vi "Waveform_Creator.vi"() -> ()   [LabVIEW 2012]
uses:
  Waveform.ctl
  Terminal_Control.vi
  <vilib>/Instr/_visa.llb/VISA Configure Serial Port (Instr).vi
panel:
  in  "COM Port":refnum<visa-resource-name>="COM3"
  in  "Terminal":i32(listbox)
  out "Active Port":refnum<visa-resource-name>
  in  "OPEN PORT":bool
  out "Waveform Library":T1[](array[typedef]) {"Envelope Shape" items=["SQUARE", "TRIANGLE", "SINE"]; "Envelope Duty Cycle" min=0.0 max=100.0 step=1.0; "Cos 1 Amplitude" min=0.0 max=100.0 step=1.0; "Cos 1 Frequency" min=0.0 max=100.0 step=0.1; "Cos 2 Amplitude" min=0.0 max=100.0 step=1.0; "Cos 2 Frequency" min=0.0 max=100.0 step=0.1}
  in  "Tab Control":enum32{"Waveform Design", "Motor Control"}(tab)
  in  "SAVE_LIBARY":bool
  in  "LOAD_LIBARY":bool
  in  "Waveform Object":T1={"Cos 2 Frequency"=2.0, "Cos 2 Amplitude"=50.0, "Cos 1 Frequency"=2.0, "Cos 1 Amplitude"=100.0, "Envelope Duty Cycle"=100.0, "Envelope Shape"=1} {"Envelope Shape" items=["SQUARE", "TRIANGLE", "SINE"]; "Envelope Duty Cycle" min=0.0 max=100.0 step=1.0; "Cos 1 Amplitude" min=0.0 max=100.0 step=1.0; "Cos 1 Frequency" min=0.0 max=100.0 step=0.1; "Cos 2 Amplitude" min=0.0 max=100.0 step=1.0; "Cos 2 Frequency" min=0.0 max=100.0 step=0.1}
  out "Waveform Graph":dbl[][](graph)
  out "Command":string="W(6,2,100,20,100,20,50)"
  in  "Program":bool
  in  "Waveform Slot":dbl=6.0 min=0.0 max=50.0 step=1.0
  in  "Run":bool[](array[boolean])=[FALSE, FALSE, FALSE, FALSE, FALSE, FALSE, TRUE, FALSE, FALSE, TRUE, FALSE, FALSE, FALSE, FALSE, FALSE, TRUE, FALSE]
  in  "Frequency_Array":dbl[](array[numeric])=[10.0, 10.0, 10.0, 10.0, 10.0, 10.0, 10.0, 10.0, 10.0, 10.0, 10.0, 10.0, 10.0, 10.0, 10.0, 10.0] caption="Frequency"
  in  "Amplitude_Array":dbl[](array[numeric])=[4095.0, 4095.0, 4095.0, 4095.0, 4095.0, 4095.0, 4095.0, 4095.0, 4095.0, 4095.0, 4095.0, 4095.0, 4095.0, 4095.0, 4095.0, 4095.0] caption="Amplitude"
  in  "Waveform Array":dbl[](array[numeric])=[0.0, 0.0, 0.0, 0.0, 0.0, 0.0, 3.0, 0.0, 0.0, 0.0, 0.0, 0.0, 0.0, 0.0, 0.0, 0.0] caption="Waveform"
  # "Amplitude"
  # "Frequency"
  # "COSINE 1"
  # "COSINE 2"
  # "Waveform Library"
  # "Amplitude"
  # "Frequency"
  # "COSINE 1"
  # "COSINE 2"
  # "Motor"
  # "1\n2\n3\n4\n5\n6\n7\n8\n9\n10\n11\n12\n13\n14\n15\n16"
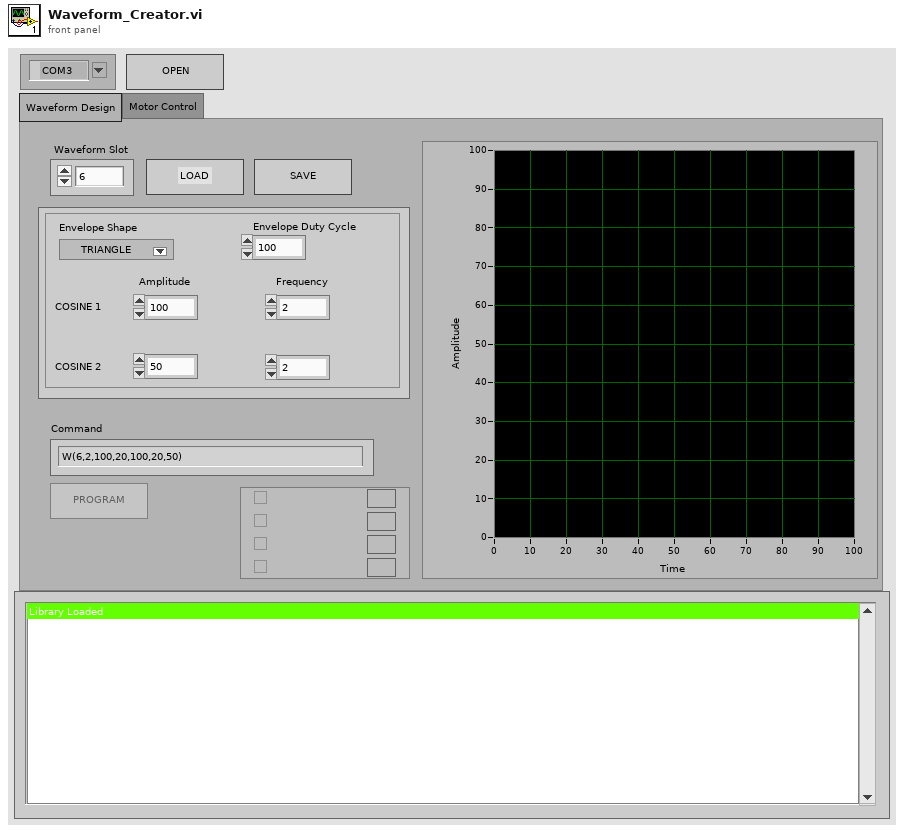
[diagram p1: front panel]
types:
  T1 = typedef "Waveform.ctl" = cluster{"Cos 2 Frequency":dbl, "Cos 2 Amplitude":dbl, "Cos 1 Frequency":dbl, "Cos 1 Amplitude":dbl, "Envelope Duty Cycle":dbl, "Envelope Shape":u16}
  T2 = enum8{"Enabled", "Disabled", "Disabled and Grayed Out"}
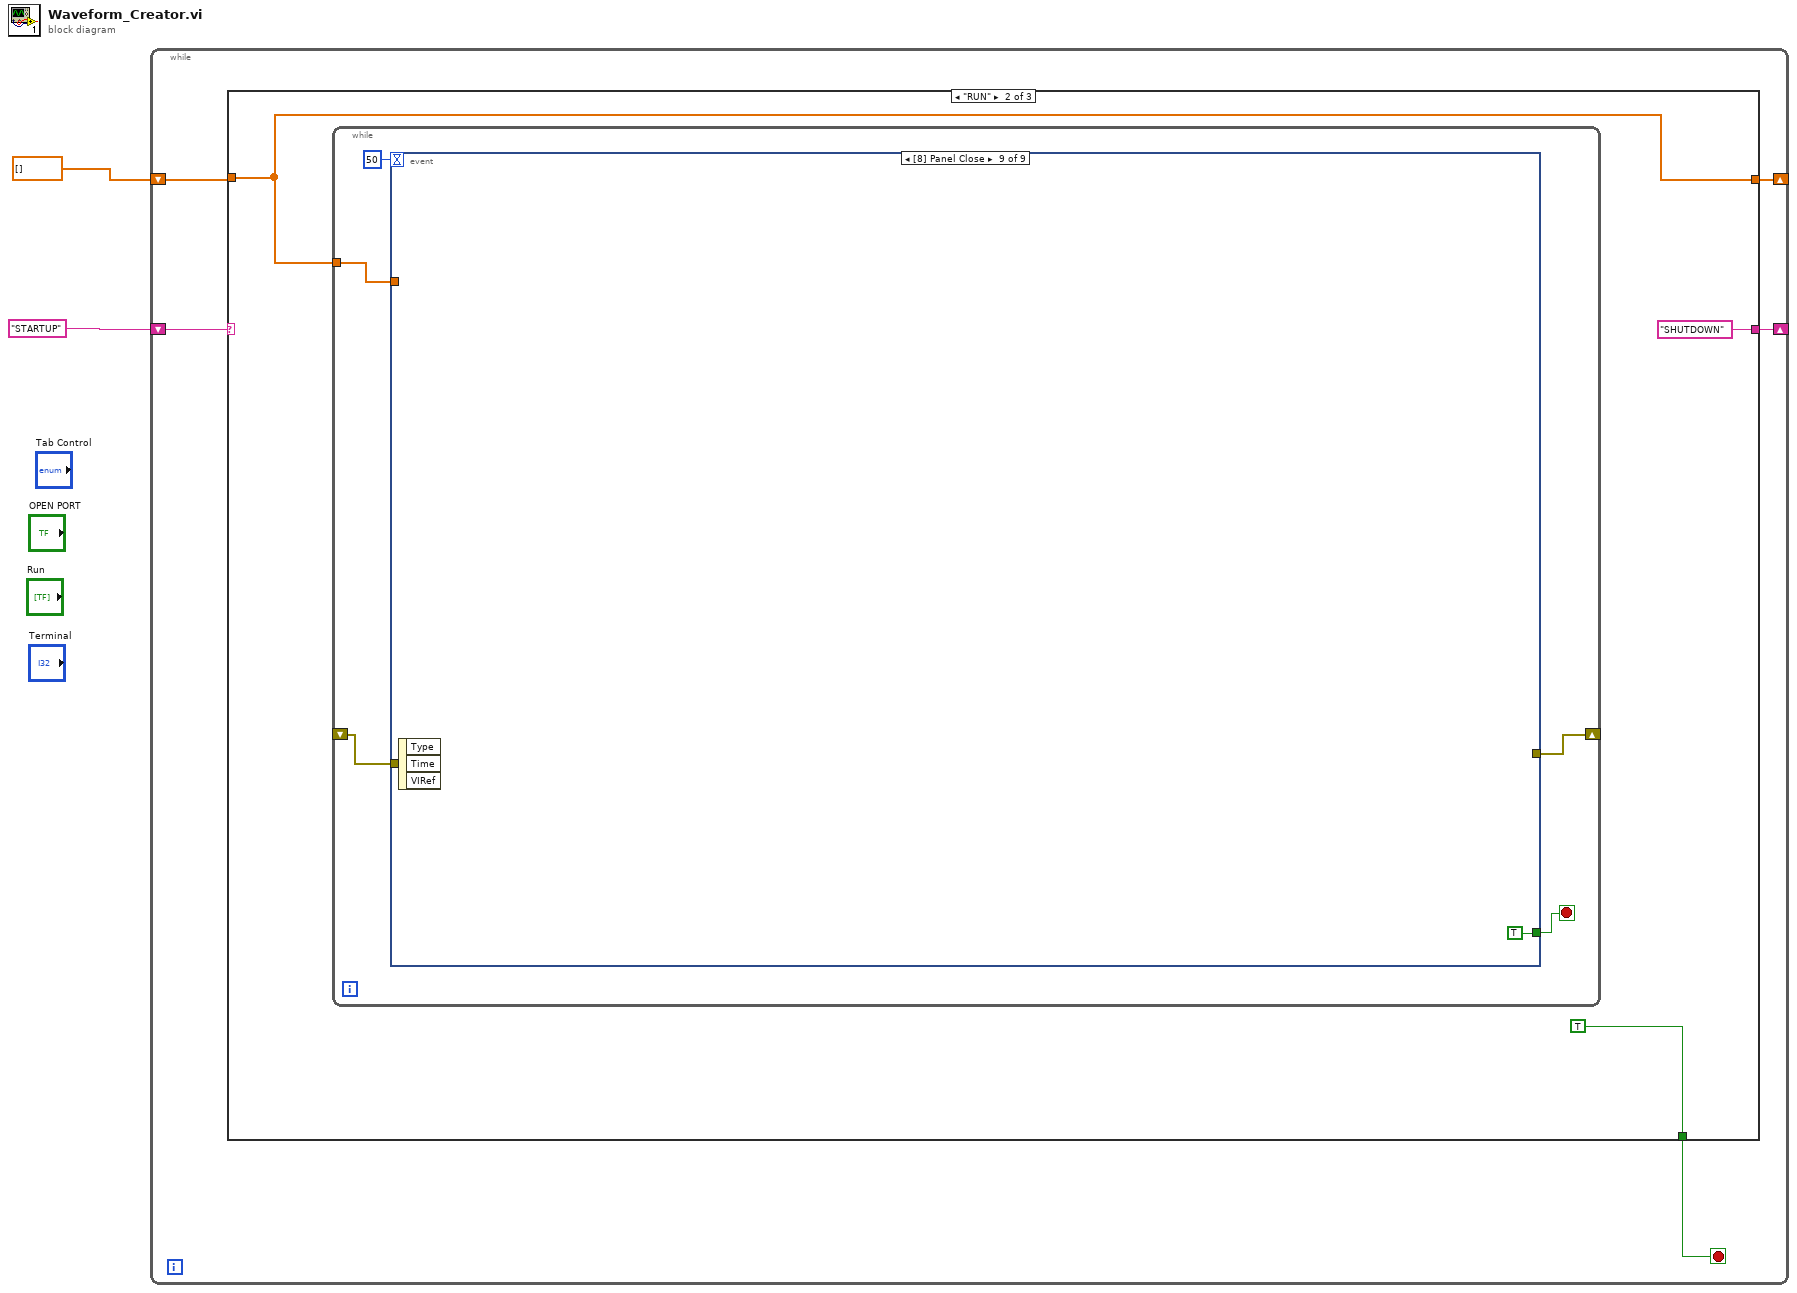
[diagram p0: block diagram]
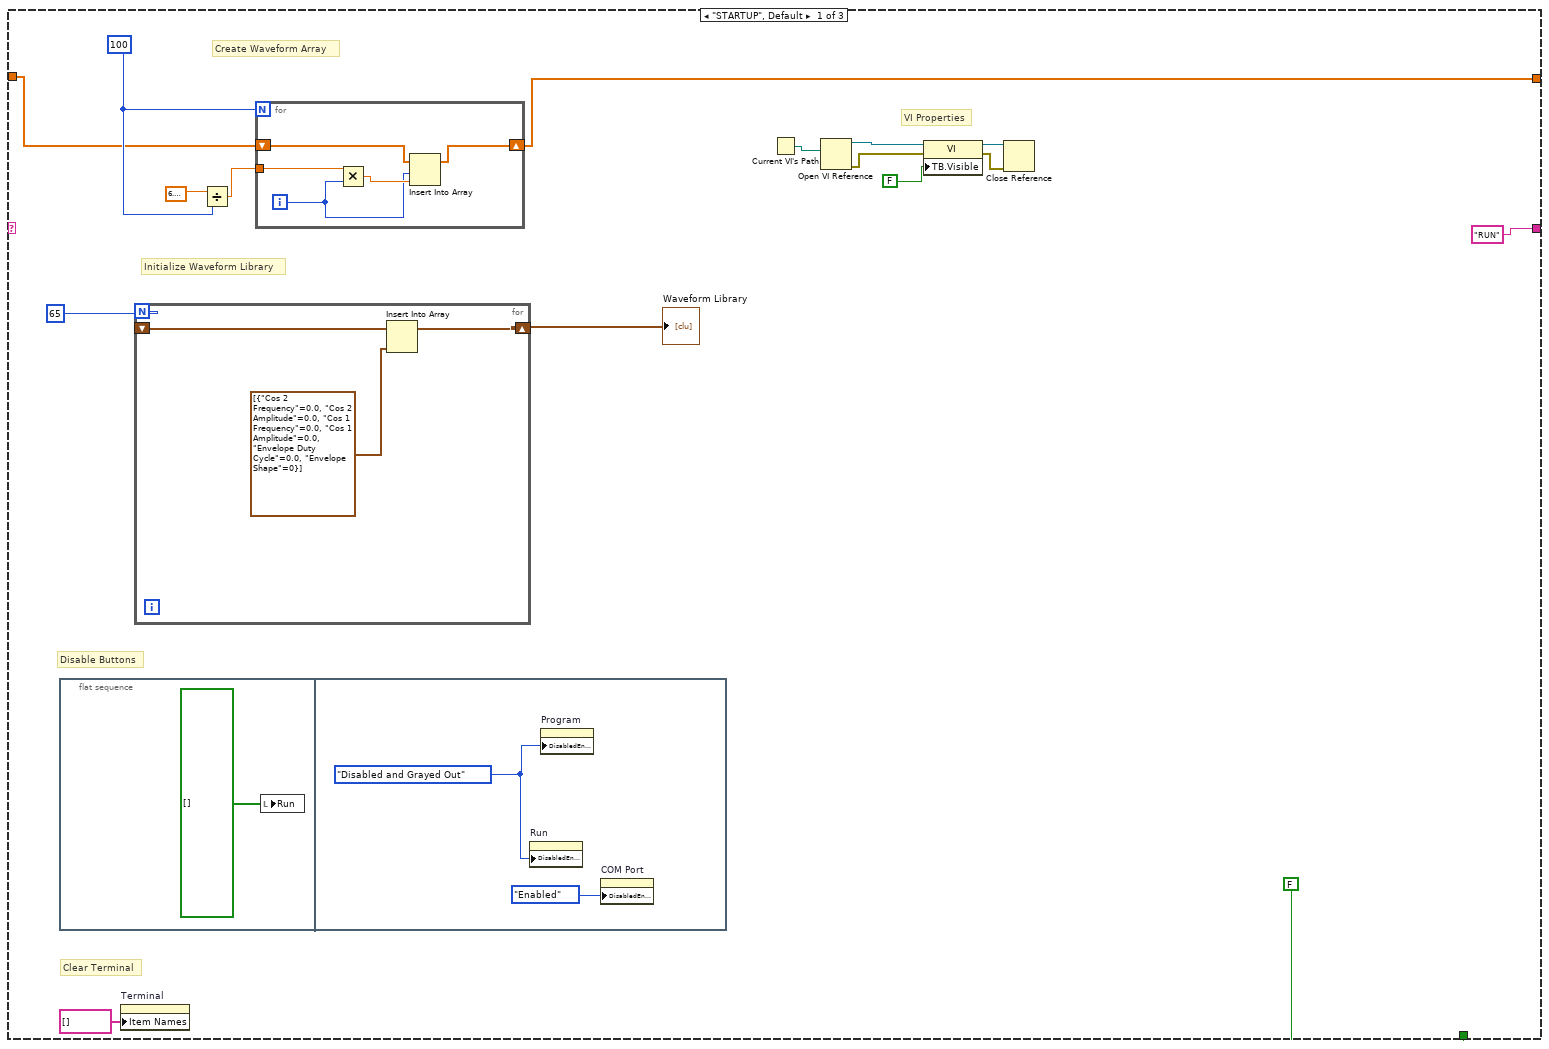
[diagram p2: hidden frame]
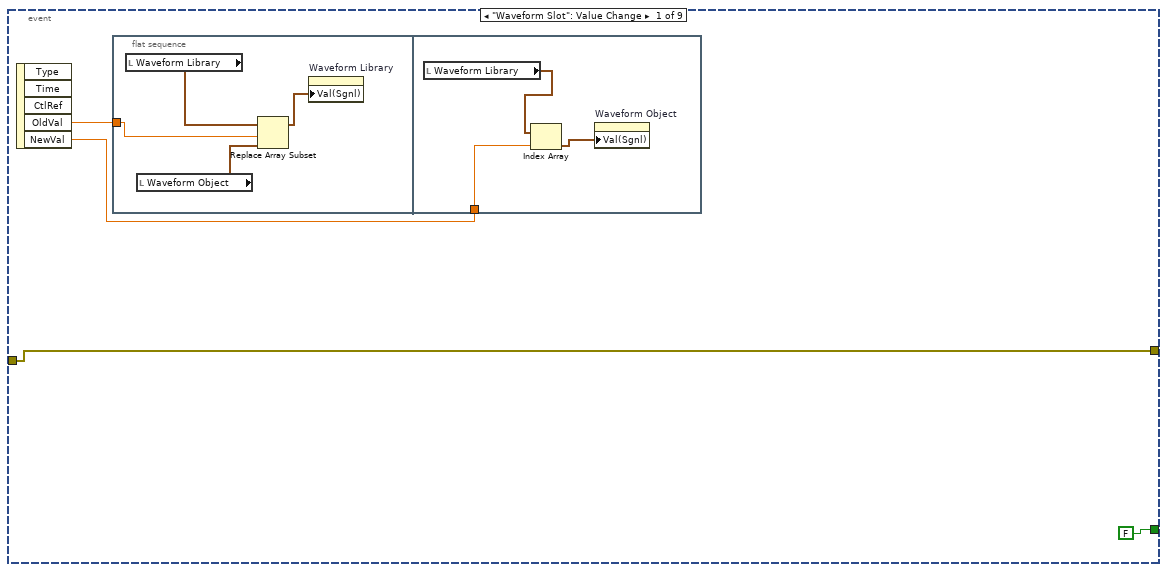
[diagram p3: hidden frame]
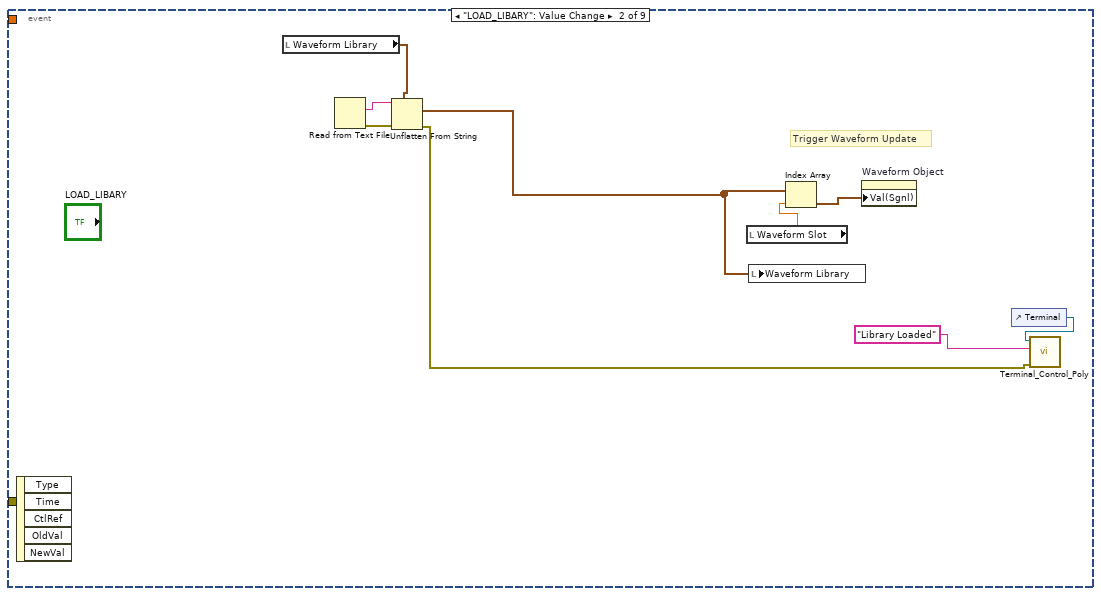
[diagram p4: hidden frame]
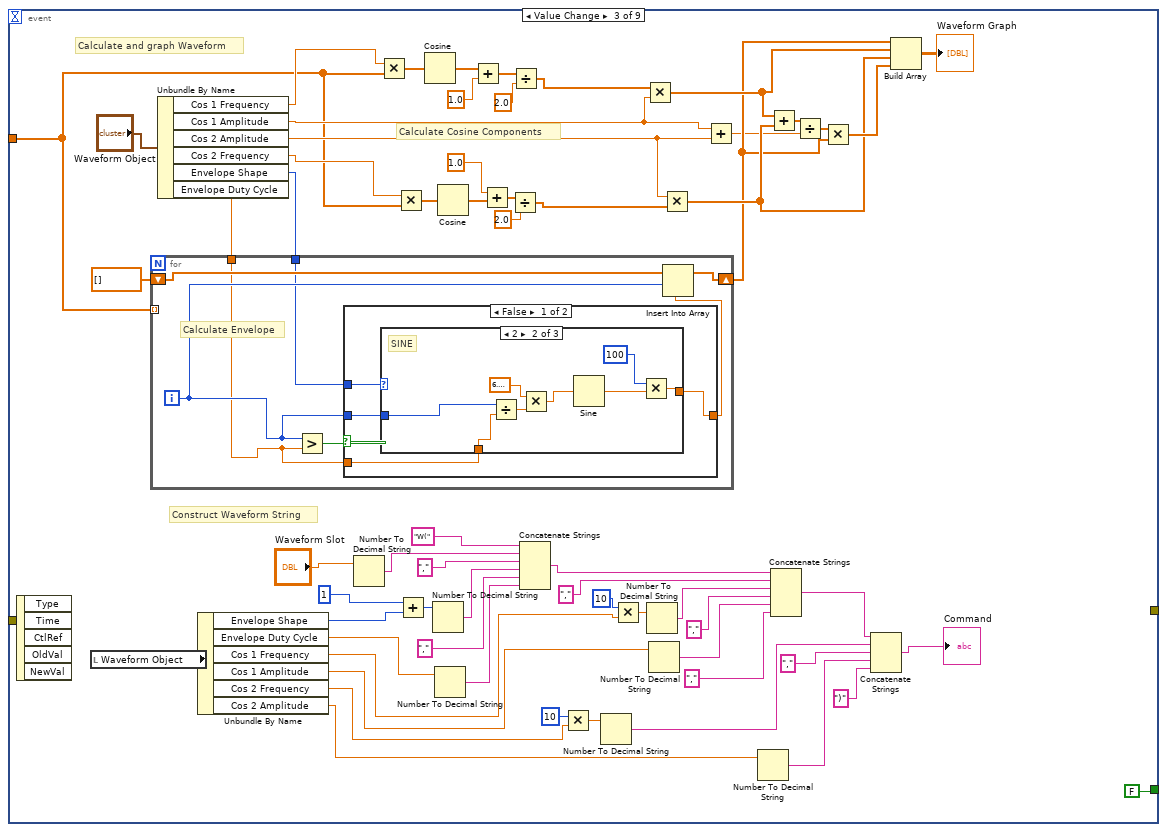
[diagram p5: hidden frame]
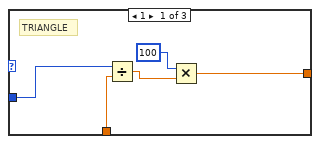
[diagram p6: hidden frame]
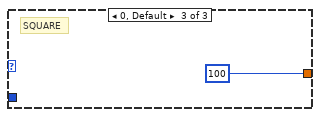
[diagram p7: hidden frame]
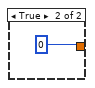
[diagram p8: hidden frame]
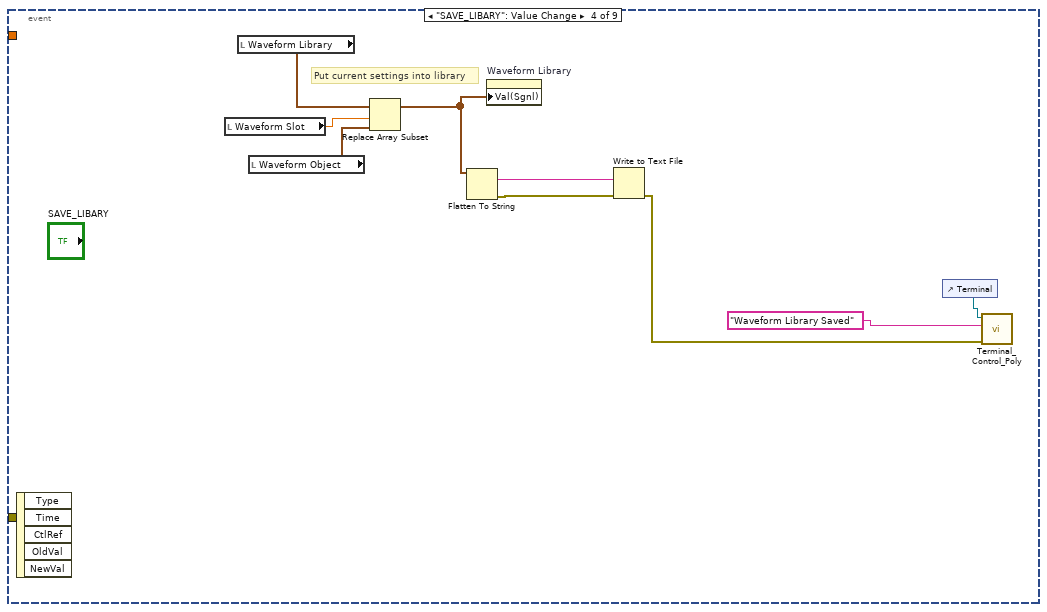
[diagram p9: hidden frame]
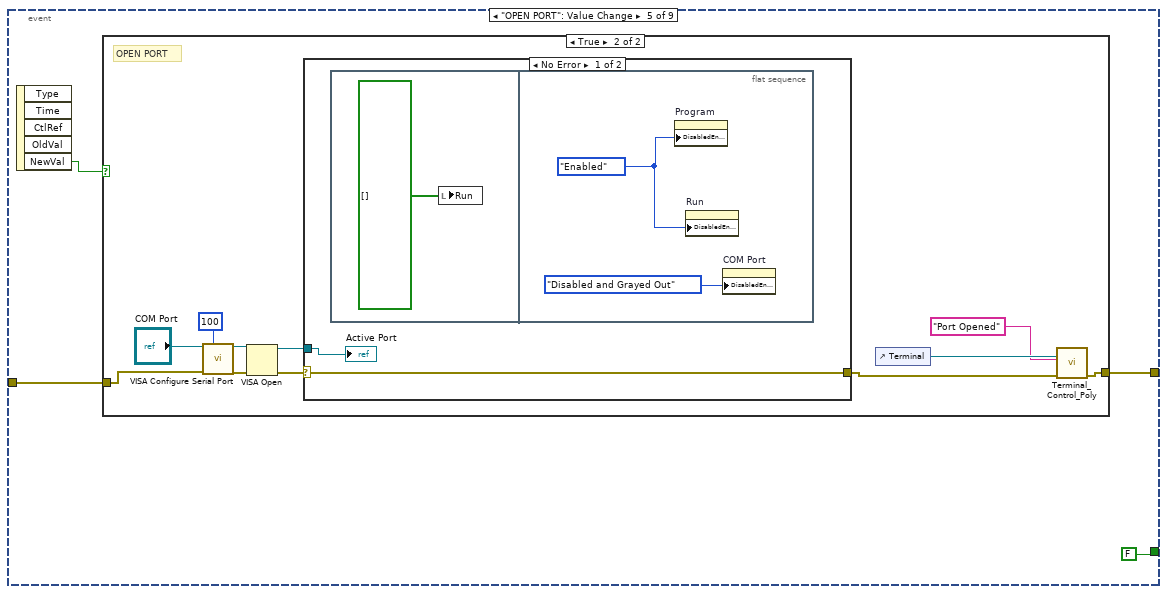
[diagram p10: hidden frame]
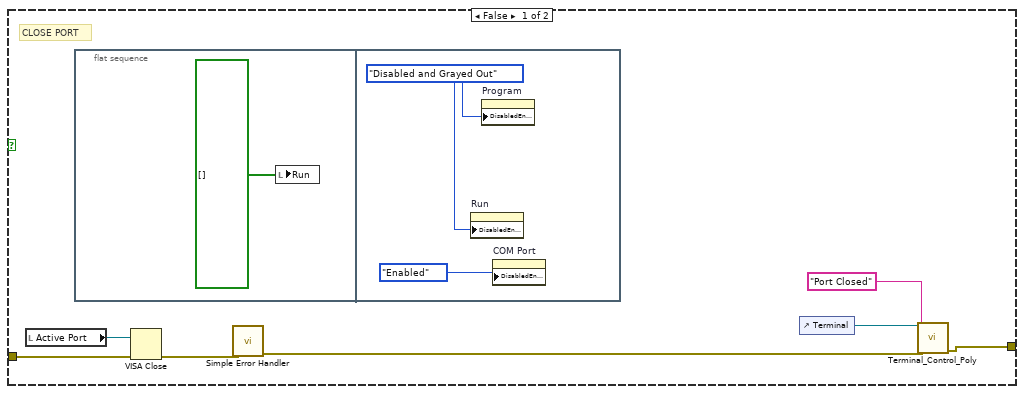
[diagram p11: hidden frame]
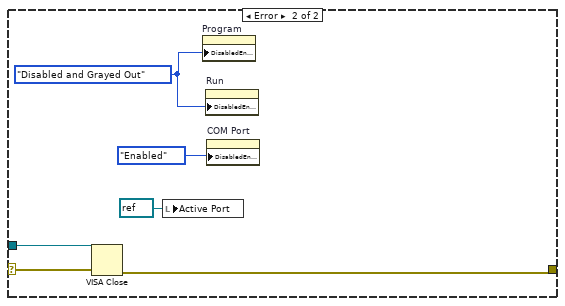
[diagram p12: hidden frame]
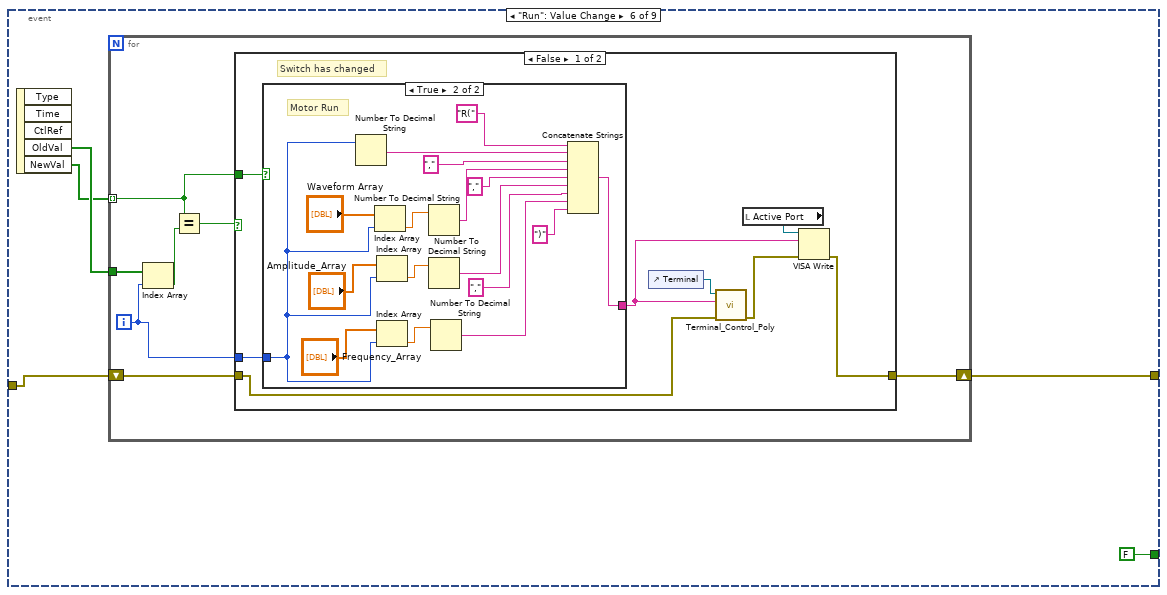
[diagram p13: hidden frame]
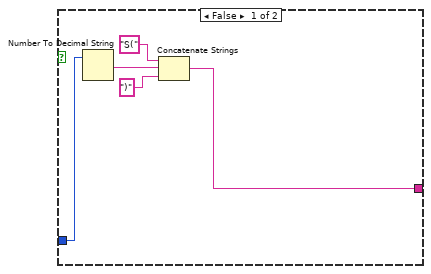
[diagram p14: hidden frame]
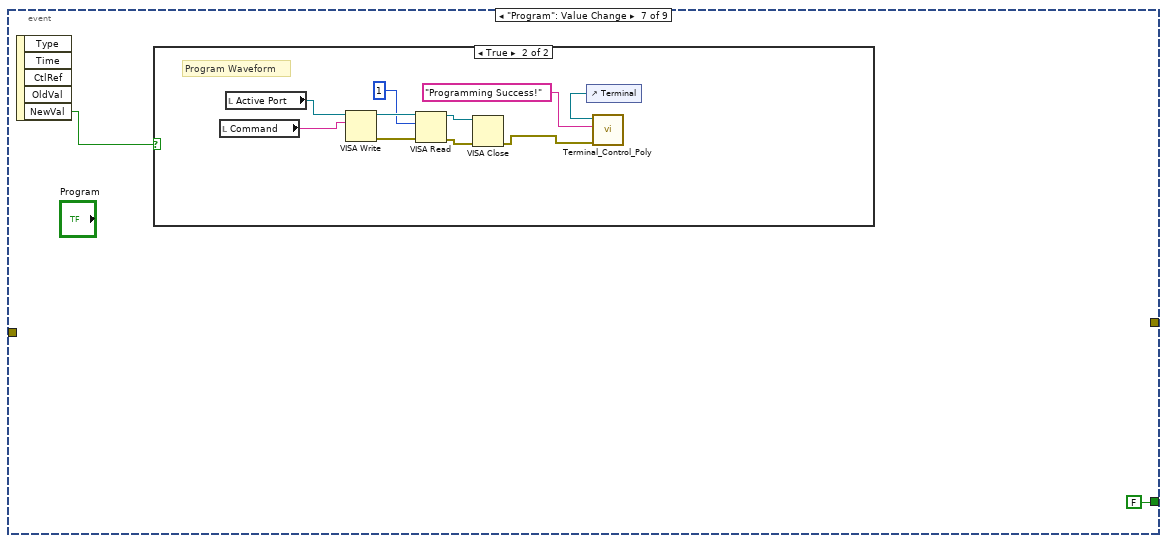
[diagram p16: hidden frame]
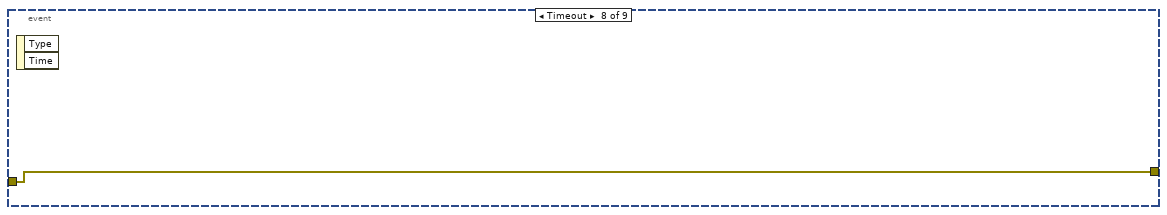
[diagram p18: hidden frame]
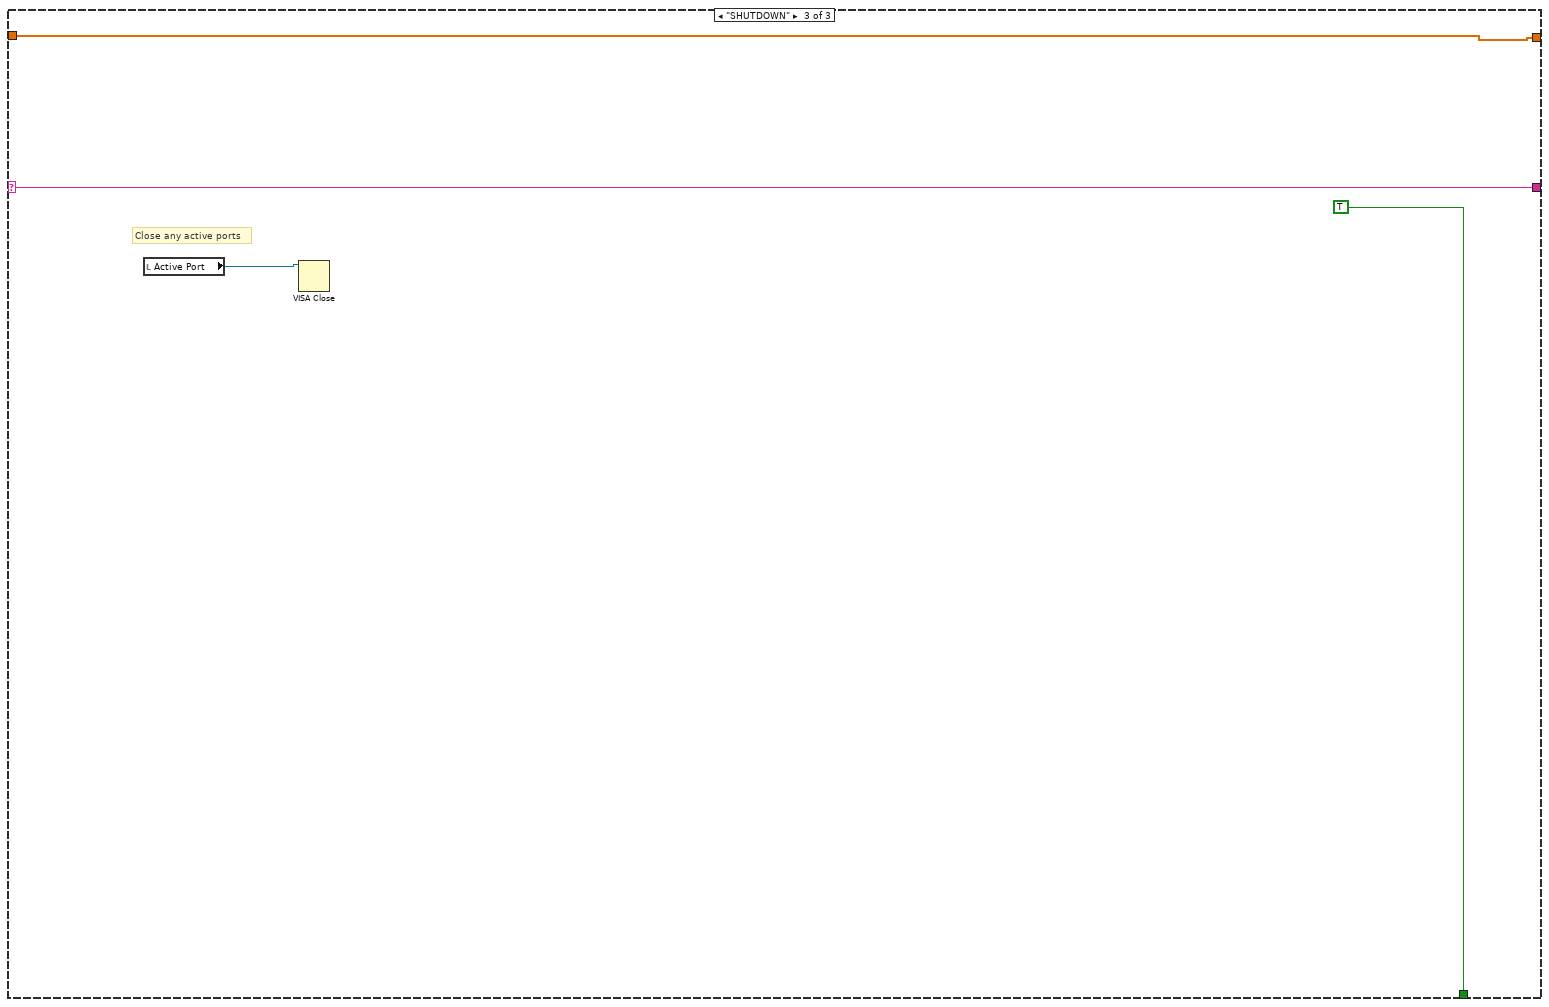
[diagram p19: hidden frame]
diagram:
  n1 = while {
    shift-right: [w4] -> _
    shift-left: "STARTUP" -> [w7]
    shift-right: [w3] -> _
    shift-left: dbl[] [] -> [w6]
    stop <- w5 stop-if-true
    n2 = case shown="\"RUN\"" w7 {
      selector: w7 -> [_ _ w253]
      tunnel: w6 -> [w14 w37 w254]
      tunnel: [FALSE TRUE TRUE] -> w5
      tunnel: ["RUN" "SHUTDOWN" w253] -> w4
      tunnel: [w16 w37 w254] -> w3
      frame "STARTUP", Default {
        w20 = 100
        # "VI Properties"
        # "Clear Terminal"
        # "Disable Buttons"
        # "Initialize Waveform Library"
        # "Create Waveform Array"
        n3 = flat-sequence {
          frame #0 {
            n4 = local write "Run"(bool[] []) -> ()
          }
          frame #1 {
            w26 = T2."Disabled and Grayed Out" ("Disabled")
            n5 = property on="Run" class="Arr (strict)"("DisabledEnum"=w26) -> ()  [unwired: 2 in, 2 out]
            n6 = property on="Program" class="Bool"("DisabledEnum"=w26) -> ()  [unwired: 2 in, 2 out]
            n7 = property on="COM Port" class="VISAName"("DisabledEnum"=T2."Enabled" ("Disabled")) -> ()  [unwired: 2 in, 2 out]
          }
        }
        n8 = property on="Terminal" class="LstBox (strict)"("Item Names"=string[] []) -> ()  [unwired: 2 in, 2 out]
        n9 = for {
          N: 65 -> [_]
          shift-right: [w33] -> w23
          shift-left: _ -> [w32]
          n10 = Insert Into Array(array=w32, new element=T1[] [{"Cos 2 Frequency"=0.0, "Cos 2 Amplitude"=0.0, "Cos 1 Frequency"=0.0, "Cos 1 Amplitude"=0.0, "Envelope Duty Cycle"=0.0, "Envelope Shape"=0}] ("Waveform Library")) -> (w33:T1[])  [unwired: 1 in]
        }
        "Waveform Library" <- w23
        n11 = Divide(x=6.283185307179586, y=w20) -> (x/y=w21:dbl)
        n12 = for {
          N: w20 -> [_]
          shift-right: [w29] -> w16
          shift-left: w14 -> [w30]
          tunnel: w21 -> [w27]
          i -> [w28]
          n13 = Multiply(x=w27, y=w28) -> (x*y=w31:dbl)
          n14 = Insert Into Array(array=w30, index=w28, new element=w31) -> (w29:dbl[])
        }
        n15 = Current VI's Path() -> (path=w13:path)
        n16 = Open VI Reference(vi path=w13) -> (vi reference=w12:refnum<vi>, error out=w11:errorcluster)  [unwired: 5 in]
        n17 = property class="VI"(reference=w12, error in=w11, "TB.Visible"=FALSE ("Tool Bar:Visible")) -> (reference out=w10:refnum<vi>, error out=w9:errorcluster)
        n18 = Close Reference(reference=w10, error in (no error)=w9) -> ()  [unwired: 1 out]
      }
      frame "RUN" {
        n19 = while {
          shift-right: [w42] -> _
          shift-left: _ -> [w41]
          tunnel: w37 -> [w40]
          stop <- w39 stop-if-true
          n20 = event shown="[8] Panel Close" {
            selector: _ -> [_ _ _ _ _ _ _ _ _]
            dyn-events: _ -> [_ _ _ _ _ _ _ _ _]
            timeout: 50 -> [_ _ _ _ _ _ _ _ _]
            tunnel: [w44 _ _ _ w162 w199 _ w251 _] -> w42
            tunnel: w41 -> [w44 _ _ _ w161 w197 _ w251 _]
            tunnel: w40 -> [_ _ w64 _ _ _ _ _ _]
            tunnel: [FALSE _ FALSE _ FALSE FALSE FALSE _ TRUE] -> w39
            event "Waveform Slot": Value Change {
              n21 = event-data() -> ("OldVal"=w45:dbl, "NewVal"=w46:dbl)  [unwired: 1 in, 3 out]
              n22 = flat-sequence {
                tunnel: w45 -> [w48]
                tunnel: w46 -> [w52]
                frame #0 {
                  n23 = local read "Waveform Library"() -> (w50:T1[])
                  n24 = local read "Waveform Object"() -> (w49:T1)
                  n25 = Replace Array Subset(array=w50, new element=w49, index=w48) -> (w47:T1[])
                  n26 = property on="Waveform Library" class="Arr (strict)"("Val(Sgnl)"=w47) -> ()  [unwired: 2 in, 2 out]
                }
                frame #1 {
                  n27 = local read "Waveform Library"() -> (w53:T1[])
                  n28 = Index Array(array=w53, index=w52) -> (element=w51:T1)
                  n29 = property on="Waveform Object" class="Clust (strict)"("Val(Sgnl)"=w51) -> ()  [unwired: 2 in, 2 out]
                }
              }
            }
            event "LOAD_LIBARY": Value Change {
              # "Trigger Waveform Update"
              n30 = event-data() -> ()  [unwired: 1 in, 5 out]
              n31 = local read "Waveform Library"() -> (w55:T1[])
              n32 = Read from Text File() -> (text=w56:string, error out=w57:errorcluster)  [unwired: 4 in, 2 out]
              n33 = Unflatten From String(type=w55, binary string=w56, error in (no error)=w57) -> (value=w54:T1[], error out=w60:errorcluster)  [unwired: 2 in, 1 out]
              n34 = local read "Waveform Slot"() -> (w58:dbl)
              n35 = local write "Waveform Library"(w54) -> ()
              n36 = Index Array(array=w54, index=w58) -> (element=w59:T1)
              n37 = property on="Waveform Object" class="Clust (strict)"("Val(Sgnl)"=w59) -> ()  [unwired: 2 in, 2 out]
              n38 = control-ref of="Terminal"() -> (w62:refnum<vi>)
              n39 = call-poly "Terminal_Control_Poly.vi"("Error In"=w60, "Text to add"="Library Loaded", "LstBox Refnum"=w62) -> ()  [unwired: 8 in, 1 out]
            }
            event Value Change {
              # "Calculate and graph Waveform"
              # "Calculate Cosine Components"
              # "Construct Waveform String"
              n40 = event-data() -> ()  [unwired: 1 in, 5 out]
              n41 = local read "Waveform Object"() -> (w124:T1)
              n42 = Unbundle By Name("Waveform Object") -> ("Cos 1 Frequency"=w70:dbl, "Cos 1 Amplitude"=w76:dbl, "Cos 2 Amplitude"=w71:dbl, "Cos 2 Frequency"=w72:dbl, "Envelope Shape"=w74:u16, "Envelope Duty Cycle"=w73:dbl)
              n43 = for {
                shift-right: [w127] -> w87
                shift-left: dbl[] [] -> [w130]
                tunnel: w73 -> [w126]
                tunnel: w74 -> [w125]
                tunnel: w64 -> [_] mode=indexing
                i -> [w128]
                # "Calculate Envelope"
                n44 = Greater?(x=w128, y=w126) -> (0:w131:bool)
                n45 = case shown="False" w131 {
                  tunnel: w128 -> [w132 _]
                  tunnel: [w134 0] -> w129
                  tunnel: w125 -> [w135 _]
                  tunnel: w126 -> [w133 _]
                  frame False {
                    n46 = case shown="2" w135 {
                      tunnel: [w136 w143 100] -> w134
                      tunnel: w133 -> [w140 w148 _]
                      tunnel: w132 -> [w139 w147 _]
                      frame 1 {
                        # "TRIANGLE"
                        n47 = Divide(x=w139, y=w140) -> (x/y=w137:dbl)
                        n48 = Multiply(x=100, y=w137) -> (x*y=w136:dbl)
                      }
                      frame 2 {
                        # "SINE"
                        n49 = Divide(x=w147, y=w148) -> (x/y=w145:dbl)
                        n50 = Multiply(x=6.283185307179586, y=w145) -> (x*y=w144:dbl)
                        n51 = Sine(x=w144) -> (sin(x)=w141:dbl)
                        n52 = Multiply(x=100, y=w141) -> (x*y=w143:dbl)
                      }
                      frame 0, Default {
                        # "SQUARE"
                      }
                    }
                  }
                  frame True {
                  }
                }
                n53 = Insert Into Array(array=w130, index=w128, new element=w129) -> (w127:dbl[])
              }
              n54 = Unbundle By Name(w124) -> ("Envelope Shape"=w118:u16, "Envelope Duty Cycle"=w119:dbl, "Cos 1 Frequency"=w120:dbl, "Cos 1 Amplitude"=w121:dbl, "Cos 2 Frequency"=w122:dbl, "Cos 2 Amplitude"=w123:dbl)
              n55 = Number To Decimal String(number="Waveform Slot") -> (decimal integer string=w115:string)  [unwired: 1 in]
              n56 = Multiply(x=w70, y=w64) -> (x*y=w65:dbl[])
              n57 = Multiply(x=w72, y=w64) -> (x*y=w66:dbl[])
              n58 = Add(x=1, y=w118) -> (x+y=w112:i32)
              n59 = Cosine(x=w65) -> (cos(x)=w78:dbl[])
              n60 = Number To Decimal String(number=w112) -> (decimal integer string=w113:string)  [unwired: 1 in]
              n61 = Number To Decimal String(number=w119) -> (decimal integer string=w109:string)  [unwired: 1 in]
              n62 = Cosine(x=w66) -> (cos(x)=w77:dbl[])
              n63 = Add(x=w78, y=1.0) -> (x+y=w81:dbl[])
              n64 = Add(x=1.0, y=w77) -> (x+y=w82:dbl[])
              n65 = Divide(x=w82, y=2.0) -> (x/y=w86:dbl[])
              n66 = Divide(x=w81, y=2.0) -> (x/y=w85:dbl[])
              n67 = Concatenate Strings("W(", w115, ",", w113, ",", w109) -> (w108:string)
              n68 = Multiply(x=10, y=w122) -> (x*y=w98:dbl)
              n69 = Number To Decimal String(number=w98) -> (decimal integer string=w100:string)  [unwired: 1 in]
              n70 = Multiply(x=10, y=w120) -> (x*y=w105:dbl)
              n71 = Multiply(x=w85, y=w76) -> (x*y=w88:dbl[])
              n72 = Number To Decimal String(number=w105) -> (decimal integer string=w106:string)  [unwired: 1 in]
              n73 = Number To Decimal String(number=w121) -> (decimal integer string=w102:string)  [unwired: 1 in]
              n74 = Multiply(x=w71, y=w86) -> (x*y=w89:dbl[])
              n75 = Add(x=w76, y=w71) -> (x+y=w68:dbl)
              n76 = Number To Decimal String(number=w123) -> (decimal integer string=w95:string)  [unwired: 1 in]
              n77 = Add(x=w88, y=w89) -> (x+y=w67:dbl[])
              n78 = Concatenate Strings(w108, ",", w106, ",", w102, ",") -> (w99:string)
              n79 = Divide(x=w67, y=w68) -> (x/y=w69:dbl[])
              n80 = Multiply(x=w69, y=w87) -> (x*y=w90:dbl[])
              n81 = Concatenate Strings(w99, w100, ",", w95, ")") -> (→"Command":string)
              n82 = Build Array(w87, w88, w89, w90) -> (→"Waveform Graph":dbl[][])
            }
            event "SAVE_LIBARY": Value Change {
              # "Put current settings into library"
              n83 = event-data() -> ()  [unwired: 1 in, 5 out]
              n84 = local read "Waveform Slot"() -> (w152:dbl)
              n85 = local read "Waveform Library"() -> (w154:T1[])
              n86 = local read "Waveform Object"() -> (w153:T1)
              n87 = Replace Array Subset(array=w154, new element=w153, index=w152) -> (w151:T1[])
              n88 = Flatten To String(anything=w151) -> (data string=w156:string, error out=w155:errorcluster)  [unwired: 3 in, 1 out]
              n89 = property on="Waveform Library" class="Arr (strict)"("Val(Sgnl)"=w151) -> ()  [unwired: 2 in, 2 out]
              n90 = Write to Text File(text=w156, error in=w155) -> (error out=w157:errorcluster)  [unwired: 2 in, 2 out]
              n91 = control-ref of="Terminal"() -> (w159:refnum<vi>)
              n92 = call-poly "Terminal_Control_Poly.vi"("Error In"=w157, "Text to add"="Waveform Library Saved", "LstBox Refnum"=w159) -> ()  [unwired: 8 in, 1 out]
            }
            event "OPEN PORT": Value Change {
              n93 = event-data() -> ("NewVal"=w163:bool)  [unwired: 1 in, 4 out]
              n94 = case shown="True" w163 {
                tunnel: [w166 w174] -> w162
                tunnel: w161 -> [w169 w178]
                frame False {
                  # "CLOSE PORT"
                  n95 = local read "Active Port"() -> (w170:refnum<visa-resource-name>)
                  n96 = flat-sequence {
                    frame #0 {
                      n97 = local write "Run"(bool[] []) -> ()
                    }
                    frame #1 {
                      w173 = T2."Disabled and Grayed Out" ("Disabled")
                      n98 = property on="Run" class="Arr (strict)"("DisabledEnum"=w173) -> ()  [unwired: 2 in, 2 out]
                      n99 = property on="Program" class="Bool"("DisabledEnum"=w173) -> ()  [unwired: 2 in, 2 out]
                      n100 = property on="COM Port" class="VISAName"("DisabledEnum"=T2."Enabled" ("Disabled")) -> ()  [unwired: 2 in, 2 out]
                    }
                  }
                  n101 = VISA Close(VISA resource name=w170, error in (no error)=w169) -> (error out=w168:errorcluster)
                  n102 = call <vilib>:"Simple Error Handler.vi"("error in (no error)"=w168) -> ("error out"=w167:errorcluster)  [unwired: 4 in, 4 out]
                  n103 = control-ref of="Terminal"() -> (w165:refnum<vi>)
                  n104 = call-poly "Terminal_Control_Poly.vi"("Error In"=w167, "Text to add"="Port Closed", "LstBox Refnum"=w165) -> ("Error Out"=w166:errorcluster)  [unwired: 8 in]
                }
                frame True {
                  # "OPEN PORT"
                  n105 = call-poly "VISA Configure Serial Port"("VISA resource name"="COM Port", "timeout (10sec)"=u32 100, "error in (no error)"=w178) -> ("VISA resource name out"=w182:refnum<visa-resource-name>, "error out"=w181:errorcluster)  [unwired: 11 in]
                  n106 = VISA Open(error in (no error)=w181, VISA resource name=w182) -> (VISA resource name=w179:refnum<visa-resource-name>, error out=w180:errorcluster)  [unwired: 3 in]
                  n107 = case shown="No Error" w180 {
                    selector: w180 -> [w185 w193]
                    tunnel: w179 -> [w186 w194]
                    tunnel: [w185 w190] -> w175
                    frame No Error {
                      n108 = flat-sequence {
                        frame #0 {
                          n109 = local write "Run"(bool[] []) -> ()
                        }
                        frame #1 {
                          w189 = T2."Enabled" ("Disabled")
                          n110 = property on="Program" class="Bool"("DisabledEnum"=w189) -> ()  [unwired: 2 in, 2 out]
                          n111 = property on="Run" class="Arr (strict)"("DisabledEnum"=w189) -> ()  [unwired: 2 in, 2 out]
                          n112 = property on="COM Port" class="VISAName"("DisabledEnum"=T2."Disabled and Grayed Out" ("Disabled")) -> ()  [unwired: 2 in, 2 out]
                        }
                      }
                      "Active Port" <- w186
                    }
                    frame Error {
                      w195 = T2."Disabled and Grayed Out" ("Disabled")
                      n113 = VISA Close(VISA resource name=w194, error in (no error)=w193) -> (error out=w190:errorcluster)
                      n114 = local write "Active Port"(refnum<visa-resource-name> refnum ("Active Port")) -> ()
                      n115 = property on="Program" class="Bool"("DisabledEnum"=w195) -> ()  [unwired: 2 in, 2 out]
                      n116 = property on="Run" class="Arr (strict)"("DisabledEnum"=w195) -> ()  [unwired: 2 in, 2 out]
                      n117 = property on="COM Port" class="VISAName"("DisabledEnum"=T2."Enabled" ("Disabled")) -> ()  [unwired: 2 in, 2 out]
                    }
                  }
                  n118 = control-ref of="Terminal"() -> (w177:refnum<vi>)
                  n119 = call-poly "Terminal_Control_Poly.vi"("Error In"=w175, "Text to add"="Port Opened", "LstBox Refnum"=w177) -> ("Error Out"=w174:errorcluster)  [unwired: 8 in]
                }
              }
            }
            event "Run": Value Change {
              n120 = event-data() -> ("OldVal"=w200:bool[], "NewVal"=w198:bool[])  [unwired: 1 in, 3 out]
              n121 = for {
                tunnel: w198 -> [w206] mode=indexing
                tunnel: w200 -> [w204]
                shift-right: [w202] -> w199
                shift-left: w197 -> [w201]
                i -> [w203]
                n122 = Index Array(array=w204, index=w203) -> (element=w205:bool)
                n123 = Equal?(x=w206, y=w205) -> (x = y?=w207:bool)
                n124 = case shown="False" w207 {
                  tunnel: w203 -> [w215 _]
                  tunnel: w206 -> [w214 _]
                  tunnel: [w209 w238] -> w202
                  tunnel: w201 -> [w208 w238]
                  frame False {
                    # "Switch has changed"
                    n125 = case shown="True" w214 {
                      tunnel: w215 -> [w217 w222]
                      tunnel: [w216 w221] -> w212
                      frame False {
                        n126 = Number To Decimal String(number=w217) -> (decimal integer string=w219:string)  [unwired: 1 in]
                        n127 = Concatenate Strings("S(", w219, ")") -> (w216:string)
                      }
                      frame True {
                        # "Motor Run"
                        n128 = Number To Decimal String(number=w222) -> (decimal integer string=w236:string)  [unwired: 1 in]
                        n129 = Index Array(array="Waveform Array", index=w222) -> (element=w233:dbl)
                        n130 = Index Array(array="Amplitude_Array", index=w222) -> (element=w229:dbl)
                        n131 = Index Array(array="Frequency_Array", index=w222) -> (element=w225:dbl)
                        n132 = Number To Decimal String(number=w233) -> (decimal integer string=w232:string)  [unwired: 1 in]
                        n133 = Number To Decimal String(number=w229) -> (decimal integer string=w228:string)  [unwired: 1 in]
                        n134 = Number To Decimal String(number=w225) -> (decimal integer string=w226:string)  [unwired: 1 in]
                        n135 = Concatenate Strings("R(", w236, ",", w232, ",", w228, ",", w226, ")") -> (w221:string)
                      }
                    }
                    n136 = control-ref of="Terminal"() -> (w210:refnum<vi>)
                    n137 = call-poly "Terminal_Control_Poly.vi"("Error In"=w208, "Text to add"=w212, "LstBox Refnum"=w210) -> ("Error Out"=w211:errorcluster)  [unwired: 8 in]
                    n138 = local read "Active Port"() -> (w213:refnum<visa-resource-name>)
                    n139 = VISA Write(VISA resource name=w213, write buffer=w212, error in (no error)=w211) -> (error out=w209:errorcluster)  [unwired: 2 out]
                  }
                  frame True {
                    # "Switch Hasn't Changed"
                  }
                }
              }
            }
            event "Program": Value Change {
              n140 = event-data() -> ("NewVal"=w240:bool)  [unwired: 1 in, 4 out]
              n141 = case shown="True" w240 {
                frame False {
                }
                frame True {
                  # "Program Waveform"
                  n142 = local read "Command"() -> (w250:string)
                  n143 = local read "Active Port"() -> (w244:refnum<visa-resource-name>)
                  n144 = VISA Write(VISA resource name=w244, write buffer=w250) -> (VISA resource name out=w249:refnum<visa-resource-name>, error out=w247:errorcluster)  [unwired: 1 in, 1 out]
                  n145 = VISA Read(VISA resource name=w249, byte count=1, error in (no error)=w247) -> (VISA resource name out=w246:refnum<visa-resource-name>, error out=w245:errorcluster)  [unwired: 2 out]
                  n146 = VISA Close(VISA resource name=w246, error in (no error)=w245) -> (error out=w243:errorcluster)
                  n147 = control-ref of="Terminal"() -> (w242:refnum<vi>)
                  n148 = call-poly "Terminal_Control_Poly.vi"("Error In"=w243, "Text to add"="Programming Success!", "LstBox Refnum"=w242) -> ()  [unwired: 8 in, 1 out]
                }
              }
            }
            event Timeout {
              n149 = event-data() -> ()  [unwired: 1 in, 2 out]
            }
            event Panel Close {
              n150 = event-data() -> ()  [unwired: 1 in, 3 out]
            }
          }
        }
      }
      frame "SHUTDOWN" {
        # "Close any active ports"
        n151 = local read "Active Port"() -> (w256:refnum<visa-resource-name>)
        n152 = VISA Close(VISA resource name=w256) -> ()  [unwired: 1 in, 1 out]
      }
    }
  }
